vi "ESTTL.vi"(8 "error in (no error)":errorcluster, 11 "Node Ptr":T4 format="%.0x") -> (0 "error out":errorcluster)   [LabVIEW 2016, in "DCM System Explorer.lvlib"]
uses:
  DCM System Explorer.lvlib
  <vilib>/NI Veristand/Custom Device API/Custom Device Item Ref.ctl
  <vilib>/Powertrain Controls/Device Drivers/DCM/ESTTL/RT/Setup.ctl
  <vilib>/Powertrain Controls/Device Drivers/DCM/ESTTL/FPGA/Mode.ctl
  <vilib>/Powertrain Controls/Device Drivers/DCM/ESTTL/RT/Angle Control.ctl
  Shared/DCM Properties.vi
  <vilib>/NI Veristand/Custom Device API/Get Item Property (String Array).vi
  Shared/DCM Constants and GUIDs.vi
  <vilib>/NI Veristand/Custom Device API/Set Item Property (String Array).vi
  <vilib>/NI VeriStand/Custom Device API/Custom Device API.lvlib
  DCM Shared.lvlib
  <vilib>/Powertrain Controls/Device Drivers/DCM/ESTTL/RT/DCM - RT - ESTTL.lvlib
  <vilib>/Powertrain Controls/Device Drivers/DCM/ESTTL/FPGA/DCM - FPGA - ESTTL.lvlib
panel:
  in  "_Setup Element":T1={"Mode"=enum."Off", "Polarity"=FALSE, "Frequency [Hz]"=0.0, "Duty Cycle [%]"=0.0, "TDC Offset [CAD]"=0.0, "Window Start [DBTDC]"=0.0, "Window End [DBTDC]"=0.0, "Angles"=[{"Enable"=FALSE, "Location [DBTDC]"=0.0, "Duration [s]"=0.0}, {"Enable"=FALSE, "Location [DBTDC]"=0.0, "Duration [s]"=0.0}, {"Enable"=FALSE, "Location [DBTDC]"=0.0, "Duration [s]"=0.0}, {"Enable"=FALSE, "Location [DBTDC]"=0.0, "Duration [s]"=0.0}], "Skip Fire"=FALSE, "Skip Fire Index"=0} {"Skip Fire Index" max=7; "Angles"."Duration [s]" format="%#_3p"; "Frequency [Hz]" format="%#_3p"}
  in  "_Refresh":bool
  in  "Channel Names":string[](array[string])=["", "", "", "", "", "", "", "", "", "", "", ""]
  in  "Channel Name":string
  in  "_ESTTL Channels":i32[](listbox) caption="Channel Summary"
  in  "_Save Changes?":bool
  in  "Setup":T1[](array[typedef]) caption="ESTTL Setup" {"Skip Fire Index" max=7; "Angles"."Duration [s]" format="%#_3p"; "Frequency [Hz]" format="%#_3p"}
  in  "Header":cluster{"Section Name":string}={"Section Name"="ESTTL I/O Initial Settings"}
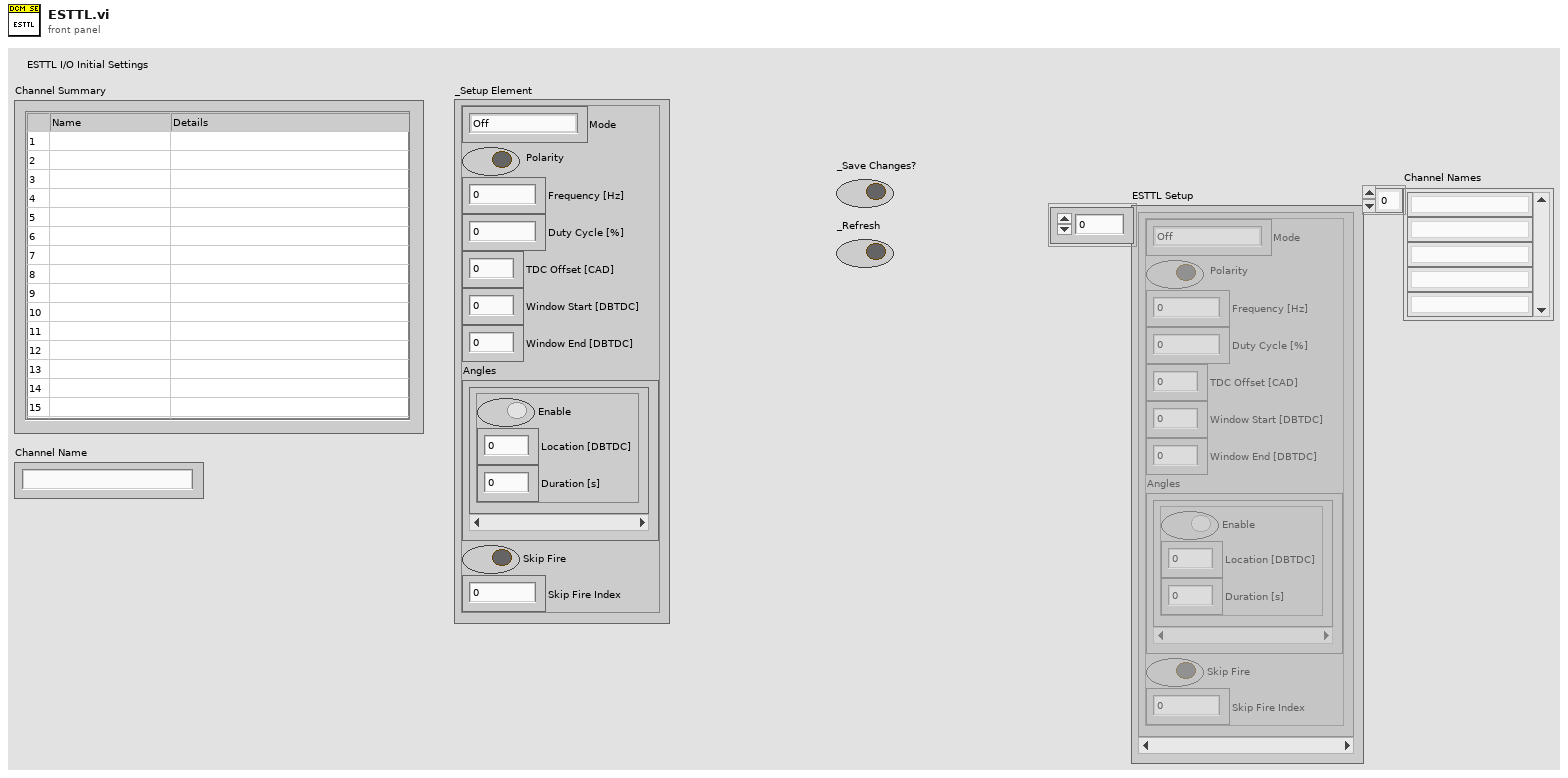
[diagram p1: front panel]
types:
  T1 = typedef "DCM - RT - ESTTL.lvlib/Setup.ctl" = cluster{"Mode":T2, "Polarity":bool, "Frequency [Hz]":sgl, "Duty Cycle [%]":sgl, "TDC Offset [CAD]":sgl, "Window Start [DBTDC]":sgl, "Window End [DBTDC]":sgl, "Angles":T3[], "Skip Fire":bool, "Skip Fire Index":u8}
  T2 = typedef "DCM - FPGA - ESTTL.lvlib/Mode.ctl" = enum8{"Off", "Pulse Width Modulation", "Engine Position Tracking"}
  T3 = typedef "DCM - RT - ESTTL.lvlib/Angle Control.ctl" = cluster{"Enable":bool, "Location [DBTDC]":sgl, "Duration [s]":sgl}
  T4 = typedef "Custom Device API.lvlib/Custom Device Item Ref.ctl" = u64
  T5 = typedef "Custom Device API.lvlib/Custom Device Commands.ctl" = enum16{"Default", "Item renamed", "Shutdown", "Dynamic button pressed"}
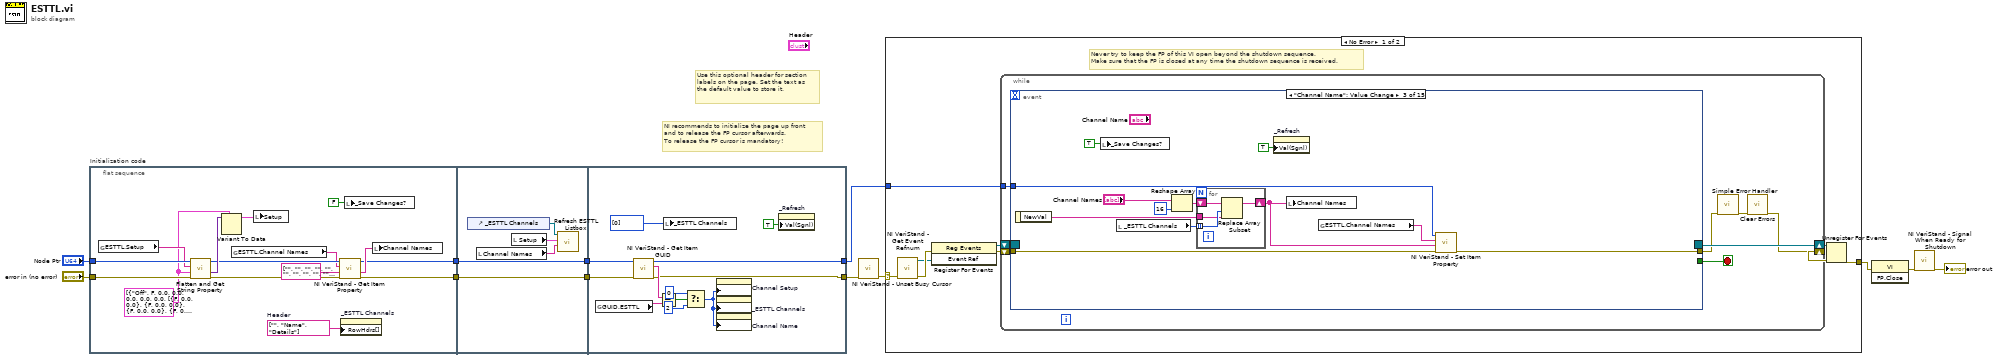
[diagram p0: block diagram]
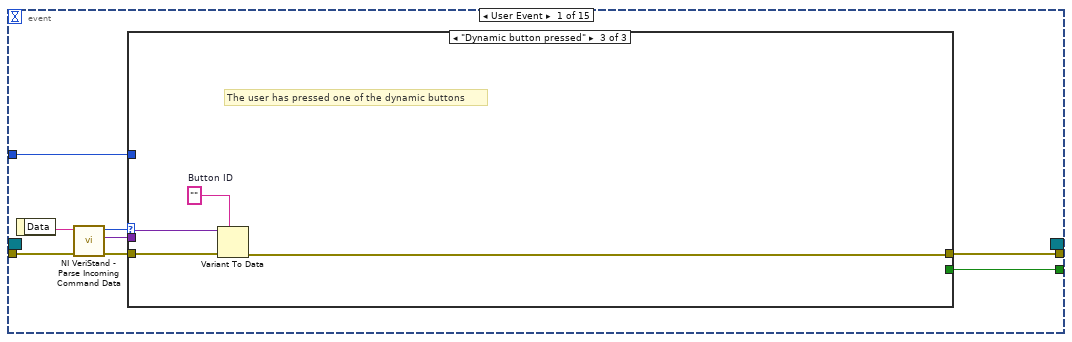
[diagram p2: hidden frame]
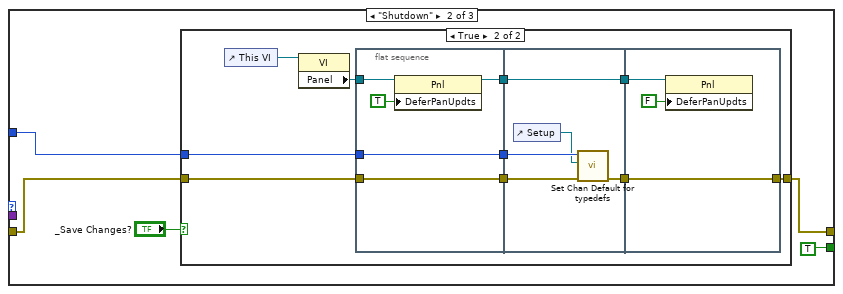
[diagram p4: hidden frame]
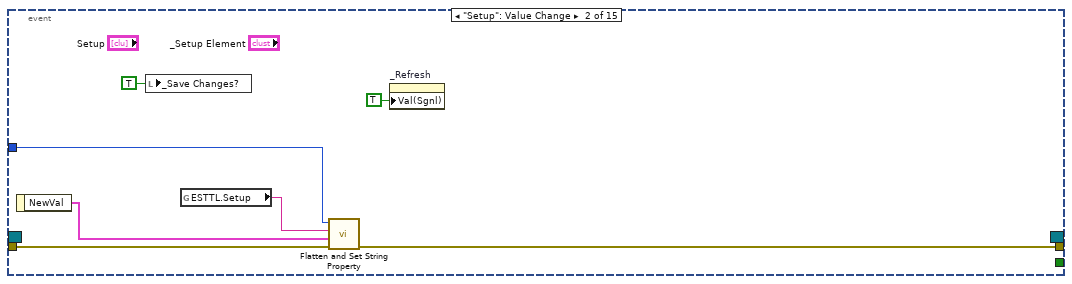
[diagram p6: hidden frame]
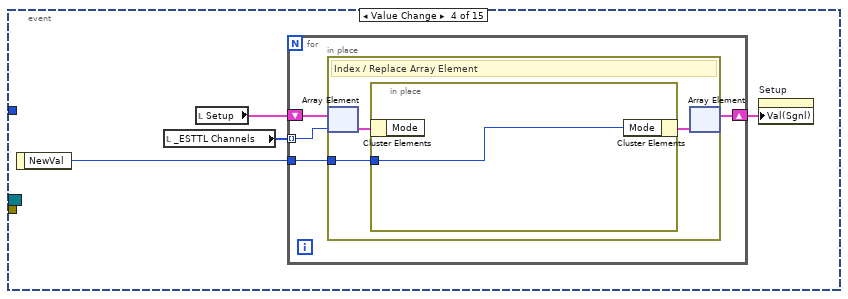
[diagram p7: hidden frame]
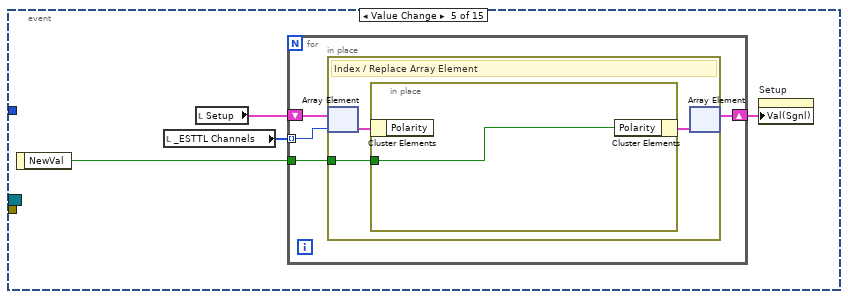
[diagram p8: hidden frame]
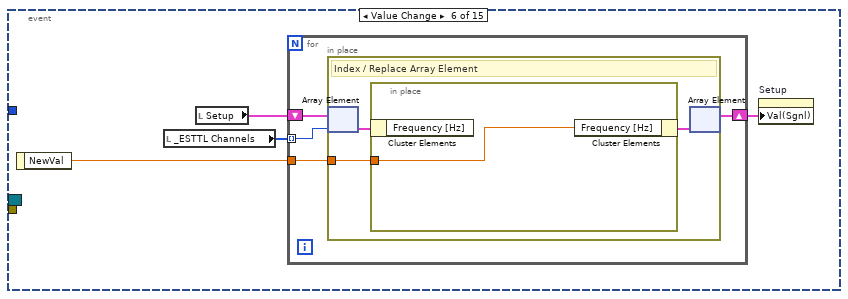
[diagram p9: hidden frame]
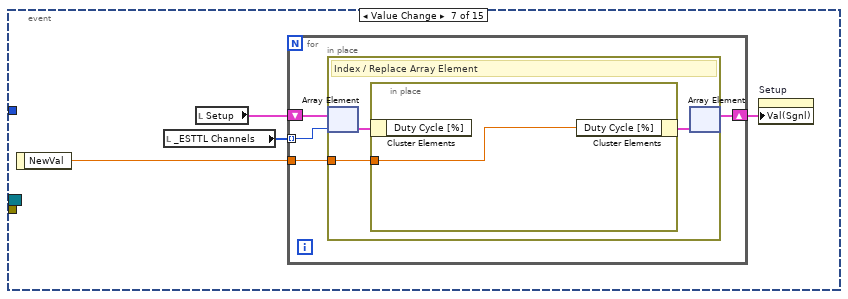
[diagram p10: hidden frame]
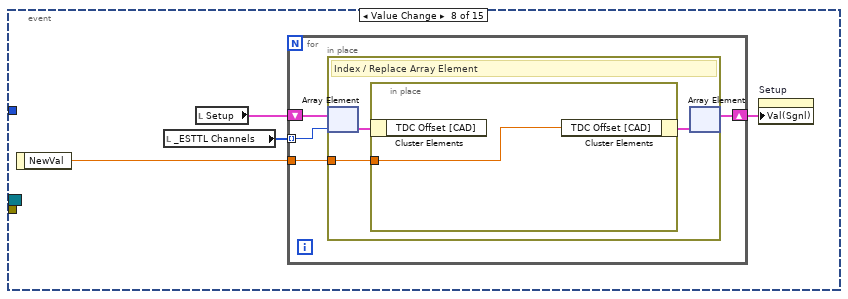
[diagram p11: hidden frame]
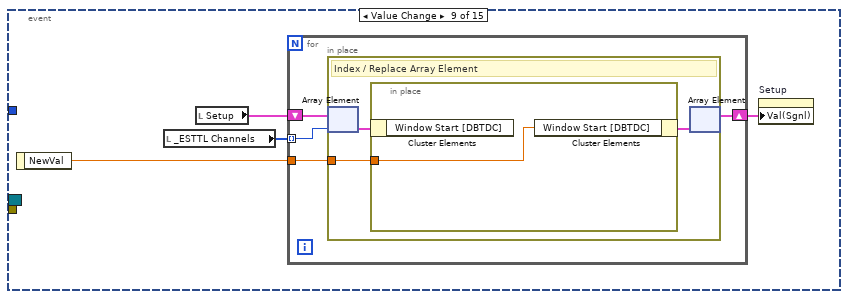
[diagram p12: hidden frame]
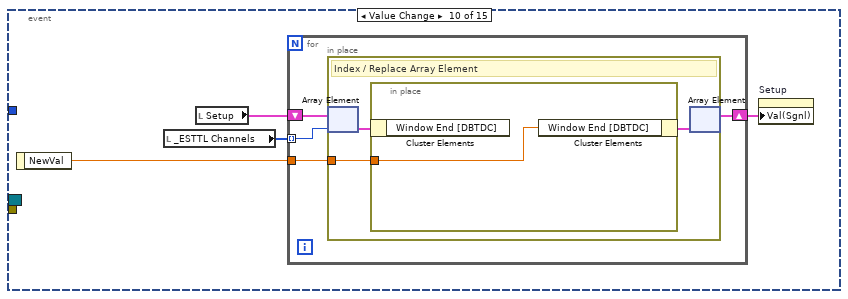
[diagram p13: hidden frame]
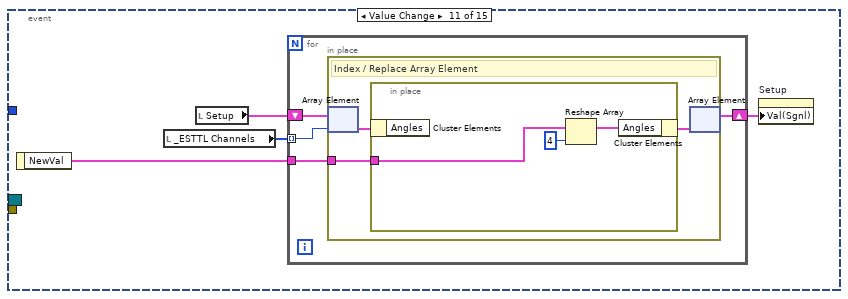
[diagram p14: hidden frame]
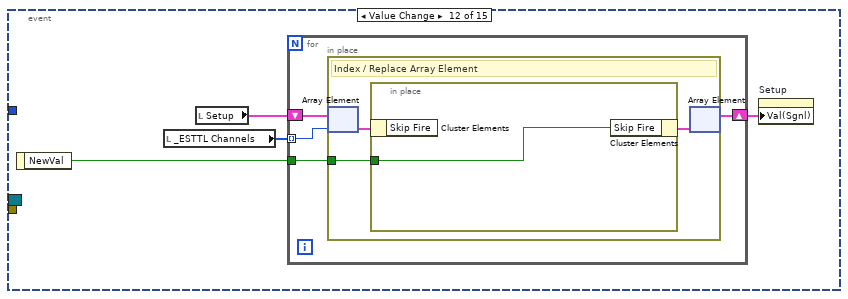
[diagram p15: hidden frame]
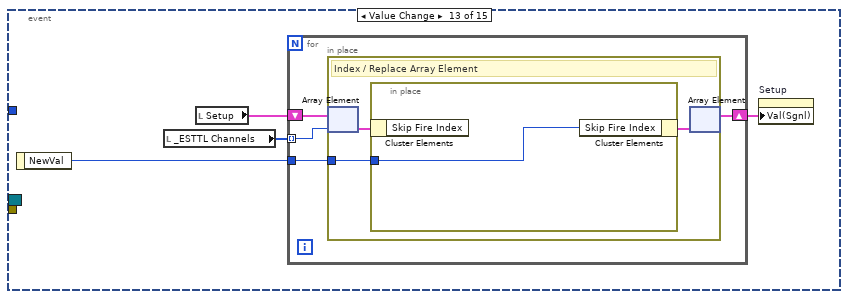
[diagram p16: hidden frame]
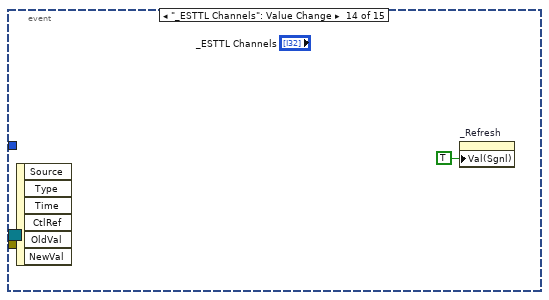
[diagram p17: hidden frame]
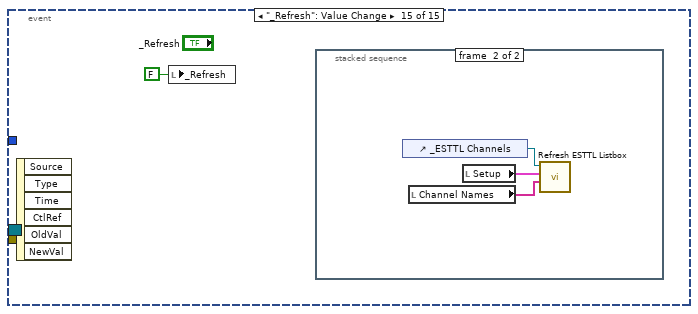
[diagram p18: hidden frame]
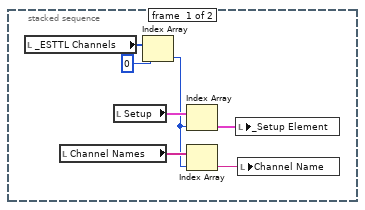
[diagram p19: hidden frame]
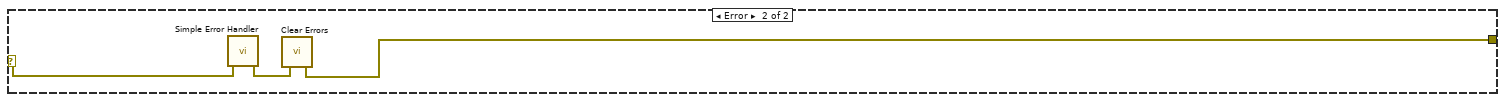
[diagram p20: hidden frame]
diagram:
  # "Use this optional header for section labels on the page. Set the text as the default value to store it."
  # "NI recommends to initialize the page up front\nand to release the FP cursor afterwards.\nTo release the FP cursor is mandatory!"
  n1 = flat-sequence "Initialization code" {
    tunnel: "Node Ptr" -> [w25]
    tunnel: "error in (no error)" -> [w26]
    tunnel: [w16] -> w5
    tunnel: [w15] -> w4
    tunnel: w5 -> [w32]
    tunnel: w4 -> [w31]
    tunnel: [w32] -> w3
    tunnel: [w31] -> w2
    tunnel: [w36] -> w1
    tunnel: [w38] -> w6
    tunnel: w3 -> [w39]
    tunnel: w2 -> [w37]
    frame #0 {
      w13 = string[] ["", "Name", "Details"]  # Header
      w23 = T1[] [{"Mode"=enum."Off", "Polarity"=FALSE, "Frequency [Hz]"=0.0, "Duty Cycle [%]"=0.0, "TDC Offset [CAD]"=0.0, "Window Start [DBTDC]"=0.0, "Window End [DBTDC]"=0.0, "Angles"=[{"Enable"=FALSE, "Location [DBTDC]"=0.0, "Duration [s]"=0.0}, {"Enable"=FALSE, "Location [DBTDC]"=0.0, "Duration [s]"=0.0}, {"Enable"=FALSE, "Location [DBTDC]"=0.0, "Duration [s]"=0.0}, {"Enable"=FALSE, "Location [DBTDC]"=0.0, "Duration [s]"=0.0}], "Skip Fire"=FALSE, "Skip Fire Index"=0}, {"Mode"=enum."Off", "Polarity"=FALSE, "Frequency [Hz]"=0.0, "Duty Cycle [%]"=0.0, "TDC Offset [CAD]"=0.0, "Window Start [DBTDC]"=0.0, "Window End [DBTDC]"=0.0, "Angles"=[{"Enable"=FALSE, "Location [DBTDC]"=0.0, "Duration [s]"=0.0}, {"Enable"=FALSE, "Location [DBTDC]"=0.0, "Duration [s]"=0.0}, {"Enable"=FALSE, "Location [DBTDC]"=0.0, "Duration [s]"=0.0}, {"Enable"=FALSE, "Location [DBTDC]"=0.0, "Duration [s]"=0.0}], "Skip Fire"=FALSE, "Skip Fire Index"=0}, {"Mode"=enum."Off", "Polarity"=FALSE, "Frequency [Hz]"=0.0, "Duty Cycle [%]"=0.0, "TDC Offset [CAD]"=0.0, "Window Start [DBTDC]"=0.0, "Window End [DBTDC]"=0.0, "Angles"=[{"Enable"=FALSE, "Location [DBTDC]"=0.0, "Duration [s]"=0.0}, {"Enable"=FALSE, "Location [DBTDC]"=0.0, "Duration [s]"=0.0}, {"Enable"=FALSE, "Location [DBTDC]"=0.0, "Duration [s]"=0.0}, {"Enable"=FALSE, "Location [DBTDC]"=0.0, "Duration [s]"=0.0}], "Skip Fire"=FALSE, "Skip Fire Index"=0}, {"Mode"=enum."Off", "Polarity"=FALSE, "Frequency [Hz]"=0.0, "Duty Cycle [%]"=0.0, "TDC Offset [CAD]"=0.0, "Window Start [DBTDC]"=0.0, "Window End [DBTDC]"=0.0, "Angles"=[{"Enable"=FALSE, "Location [DBTDC]"=0.0, "Duration [s]"=0.0}, {"Enable"=FALSE, "Location [DBTDC]"=0.0, "Duration [s]"=0.0}, {"Enable"=FALSE, "Location [DBTDC]"=0.0, "Duration [s]"=0.0}, {"Enable"=FALSE, "Location [DBTDC]"=0.0, "Duration [s]"=0.0}], "Skip Fire"=FALSE, "Skip Fire Index"=0}, {"Mode"=enum."Off", "Polarity"=FALSE, "Frequency [Hz]"=0.0, "Duty Cycle [%]"=0.0, "TDC Offset [CAD]"=0.0, "Window Start [DBTDC]"=0.0, "Window End [DBTDC]"=0.0, "Angles"=[{"Enable"=FALSE, "Location [DBTDC]"=0.0, "Duration [s]"=0.0}, {"Enable"=FALSE, "Location [DBTDC]"=0.0, "Duration [s]"=0.0}, {"Enable"=FALSE, "Location [DBTDC]"=0.0, "Duration [s]"=0.0}, {"Enable"=FALSE, "Location [DBTDC]"=0.0, "Duration [s]"=0.0}], "Skip Fire"=FALSE, "Skip Fire Index"=0}, {"Mode"=enum."Off", "Polarity"=FALSE, "Frequency [Hz]"=0.0, "Duty Cycle [%]"=0.0, "TDC Offset [CAD]"=0.0, "Window Start [DBTDC]"=0.0, "Window End [DBTDC]"=0.0, "Angles"=[{"Enable"=FALSE, "Location [DBTDC]"=0.0, "Duration [s]"=0.0}, {"Enable"=FALSE, "Location [DBTDC]"=0.0, "Duration [s]"=0.0}, {"Enable"=FALSE, "Location [DBTDC]"=0.0, "Duration [s]"=0.0}, {"Enable"=FALSE, "Location [DBTDC]"=0.0, "Duration [s]"=0.0}], "Skip Fire"=FALSE, "Skip Fire Index"=0}, {"Mode"=enum."Off", "Polarity"=FALSE, "Frequency [Hz]"=0.0, "Duty Cycle [%]"=0.0, "TDC Offset [CAD]"=0.0, "Window Start [DBTDC]"=0.0, "Window End [DBTDC]"=0.0, "Angles"=[{"Enable"=FALSE, "Location [DBTDC]"=0.0, "Duration [s]"=0.0}, {"Enable"=FALSE, "Location [DBTDC]"=0.0, "Duration [s]"=0.0}, {"Enable"=FALSE, "Location [DBTDC]"=0.0, "Duration [s]"=0.0}, {"Enable"=FALSE, "Location [DBTDC]"=0.0, "Duration [s]"=0.0}], "Skip Fire"=FALSE, "Skip Fire Index"=0}, {"Mode"=enum."Off", "Polarity"=FALSE, "Frequency [Hz]"=0.0, "Duty Cycle [%]"=0.0, "TDC Offset [CAD]"=0.0, "Window Start [DBTDC]"=0.0, "Window End [DBTDC]"=0.0, "Angles"=[{"Enable"=FALSE, "Location [DBTDC]"=0.0, "Duration [s]"=0.0}, {"Enable"=FALSE, "Location [DBTDC]"=0.0, "Duration [s]"=0.0}, {"Enable"=FALSE, "Location [DBTDC]"=0.0, "Duration [s]"=0.0}, {"Enable"=FALSE, "Location [DBTDC]"=0.0, "Duration [s]"=0.0}], "Skip Fire"=FALSE, "Skip Fire Index"=0}] ("DiffIO.Setup")
      n2 = global read "DCM Properties.vi" "ESTTL.Setup"() -> (w24:string)
      n3 = call "Flatten and Get String Property.vi"("error in (no error)"=w26, "Default Value"=w23, "Property Name"=w24, "Section Ref in"=w25) -> ("error out"=w20:errorcluster, "Value"=w27:variant, "Section Ref out"=w21:T4)  [unwired: 5 in]
      n4 = Variant To Data(type=w23, Variant=w27) -> (data=w22:T1[])  [unwired: 1 in, 1 out]
      n5 = global read "DCM Properties.vi" "ESTTL.Channel Names"() -> (w18:string)
      n6 = local write "Setup"(w22) -> ()
      n7 = call-poly <vilib>:"NI VeriStand - Get Item Property.vi"("error in (no error)"=w20, "Default Value"=string[] ["", "", "", "", "", "", "", "", "", "", "", "", "", "", "", ""], "Property Name"=w18, "Item Ref in"=w21) -> ("error out"=w15:errorcluster, "Value"=w17:string[], "Item Ref out"=w16:T4)  [unwired: 4 in, 1 out]
      n8 = property on="_ESTTL Channels" class="MCListbox (strict)"("RowHdrs[]"=w13) -> ()  [unwired: 2 in, 2 out]
      n9 = local write "_Save Changes?"(FALSE ("_Save Changes?")) -> ()
      n10 = local write "Channel Names"(w17) -> ()
    }
    frame #1 {
      n11 = control-ref of="_ESTTL Channels"() -> (w28:refnum<vi>)
      n12 = local read "Channel Names"() -> (w30:string[])
      n13 = local read "Setup"() -> (w29:T1[])
      n14 = call "Refresh ESTTL Listbox.vi"("Names"=w30, "Setup"=w29, "MulticolumnListbox in"=w28) -> ()  [unwired: 9 in]
    }
    frame #2 {
      n15 = global read "DCM Constants and GUIDs.vi" "GUID.ESTTL"() -> (w40:string)
      n16 = call <vilib>:"NI VeriStand - Get Item GUID.vi"("error in (no error)"=w37, "Item Ref in"=w39) -> ("error out"=w36:errorcluster, "GUID"=w41:string, "Item Ref out"=w38:T4)  [unwired: 7 in]
      n17 = Equal?(x=w41, y=w40) -> (x = y?=w35:bool)
      n18 = local write "_ESTTL Channels"(i32[] [0] ("Channel Setup Summary")) -> ()
      n19 = Select(t=0, s=w35, f=2) -> (s? t:f=w44:i32)
      n20 = property on="Channel Setup" class="Clust (strict)"("DisabledEnum"=w44) -> ()  [unwired: 2 in, 2 out]
      n21 = property on="_ESTTL Channels" class="MCListbox (strict)"("DisabledEnum"=w44) -> ()  [unwired: 2 in, 2 out]
      n22 = property on="Channel Name" class="Str"("DisabledEnum"=w44) -> ()  [unwired: 2 in, 2 out]
      n23 = property on="_Refresh" class="Bool (strict)"("Val(Sgnl)"=TRUE ("_Refresh")) -> ()  [unwired: 2 in, 2 out]
    }
  }
  n24 = call <vilib>:"NI VeriStand - Unset Busy Cursor.vi"("error in (no error)"=w1) -> ("error out"=w8:errorcluster)  [unwired: 10 out]
  n25 = case shown="No Error" w8 {
    selector: w8 -> [w46 w263]
    tunnel: [w50 w261] -> w12
    tunnel: w6 -> [w45 _]
    frame No Error {
      # "Never try to keep the FP of this VI open beyond the shutdown sequence.\nMake sure that the FP is closed at any time the shutdown sequence is received."
      n26 = call <vilib>:"NI VeriStand - Get Event Refnum.vi"("error in (no error)"=w46) -> ("error out"=w53:errorcluster, "Event Ref"=w49:refnum<user-event>)  [unwired: 9 out]
      n27 = register-events(error in=w53, w49) -> (reference out=w47:refnum<event-registration>, error out=w48:errorcluster)  [unwired: 1 in]
      n28 = while {
        shift-right: [w55] -> w51
        shift-left: w48 -> [w60]
        shift-right: [w61] -> w52
        shift-left: w47 -> [w59]
        tunnel: w45 -> [w54]
        stop <- w58 stop-if-true
        n29 = event shown="[2] \"Channel Name\": Value Change" {
          selector: w59 -> [_ _ _ _ _ _ _ _ _ _ _ _ _ _ _]
          dyn-events: [_ _ _ _ _ _ _ _ _ _ _ _ _ _ _] -> w61
          timeout: _ -> [_ _ _ _ _ _ _ _ _ _ _ _ _ _ _]
          tunnel: w60 -> [w69 w110 w122 _ _ _ _ _ _ _ _ _ _ _ _]
          tunnel: [w65 _ _ _ _ _ _ _ _ _ _ _ _ _ _] -> w58
          tunnel: [w64 w109 w121 _ _ _ _ _ _ _ _ _ _ _ _] -> w57
          tunnel: w54 -> [w62 w106 w119 _ _ _ _ _ _ _ _ _ _ _ _]
          event User Event {
            n30 = event-data() -> ("Data"=w68:string)  [unwired: 1 out]
            n31 = call <vilib>:"NI VeriStand - Parse Incoming Command Data.vi"("error in (no error)"=w69, "Incoming data"=w68) -> ("error out"=w67:errorcluster, "Outgoing data"=w63:variant, "Action"=w66:T5)  [unwired: 7 out]
            n32 = case shown="\"Dynamic button pressed\"" w66 {
              tunnel: w67 -> [w70 w73 w103]
              tunnel: [_ TRUE _] -> w65
              tunnel: [w70 w72 w100] -> w64
              tunnel: w63 -> [_ _ w102]
              tunnel: w62 -> [_ w74 _]
              frame "Default", Default {
              }
              frame "Shutdown" {
                n33 = case shown="True" "_Save Changes?" {
                  tunnel: w74 -> [_ w81]
                  tunnel: w73 -> [w76 w80]
                  tunnel: [w76 w79] -> w72
                  frame False {
                  }
                  frame True {
                    n34 = control-ref of="This VI"() -> (w78:refnum<vi>)
                    n35 = property class="VI"(reference=w78) -> ("Panel"=w77:refnum<vi>)  [unwired: 1 in, 2 out]
                    n36 = flat-sequence {
                      tunnel: w80 -> [w90]
                      tunnel: w81 -> [w91]
                      tunnel: [w91] -> w86
                      tunnel: [w90] -> w85
                      tunnel: w77 -> [w89]
                      tunnel: [w87] -> w84
                      tunnel: w86 -> [w96]
                      tunnel: w85 -> [w95]
                      tunnel: [w94] -> w83
                      tunnel: [w93] -> w82
                      tunnel: w84 -> [w93]
                      tunnel: [w99] -> w79
                      tunnel: w83 -> [w99]
                      tunnel: w82 -> [w97]
                      frame #0 {
                        n37 = property class="Pnl"(reference=w89, "DeferPanUpdts"=TRUE ("Defer Panel Updates")) -> (reference out=w87:refnum<vi>)  [unwired: 1 in, 1 out]
                      }
                      frame #1 {
                        n38 = control-ref of="Setup"() -> (w92:refnum<vi>)
                        n39 = call "Set Chan Default for typedefs.vi"("error in"=w95, "Ctl Ref"=w92, "Section Ref in"=w96) -> ("error out"=w94:errorcluster)  [unwired: 7 in, 1 out]
                      }
                      frame #2 {
                        n40 = property class="Pnl"(reference=w97, "DeferPanUpdts"=FALSE ("Defer Panel Updates")) -> ()  [unwired: 1 in, 2 out]
                      }
                    }
                  }
                }
              }
              frame "Dynamic button pressed" {
                w101 = ""  # Button ID
                # "The user has pressed one of the dynamic buttons"
                n41 = Variant To Data(error in=w103, type=w101, Variant=w102) -> (error out=w100:errorcluster)  [unwired: 1 out]
              }
            }
          }
          event "Setup": Value Change {
            n42 = event-data() -> ("NewVal"=w107:T1[])  [unwired: 1 out]
            n43 = local write "_Save Changes?"(TRUE ("_Save Changes?")) -> ()
            n44 = global read "DCM Properties.vi" "ESTTL.Setup"() -> (w108:string)
            n45 = call "Flatten and Set String Property.vi"("error in (no error)"=w110, "Value"=w107, "Property Name"=w108, "Section Ref in"=w106) -> ("error out"=w109:errorcluster)  [unwired: 6 in, 1 out]
            n46 = property on="_Refresh" class="Bool (strict)"("Val(Sgnl)"=TRUE ("_Refresh")) -> ()  [unwired: 2 in, 2 out]
          }
          event "Channel Name": Value Change {
            n47 = event-data() -> ("NewVal"=w113:string)  [unwired: 1 out]
            n48 = local write "_Save Changes?"(TRUE ("_Save Changes?")) -> ()
            n49 = local read "_ESTTL Channels"() -> (w115:i32[])
            n50 = Reshape Array("Channel Names", 16 ("dimension size")) -> (w117:string[])
            n51 = for {
              tunnel: w115 -> [w124] mode=indexing
              shift-right: [w125] -> w111
              shift-left: w117 -> [w126]
              tunnel: w113 -> [w123]
              n52 = Replace Array Subset(array=w126, new element=w123, index=w124) -> (w125:string[])
            }
            n53 = property on="_Refresh" class="Bool (strict)"("Val(Sgnl)"=TRUE ("_Refresh")) -> ()  [unwired: 2 in, 2 out]
            n54 = local write "Channel Names"(w111) -> ()
            n55 = global read "DCM Properties.vi" "ESTTL.Channel Names"() -> (w120:string)
            n56 = call-poly <vilib>:"NI VeriStand - Set Item Property.vi"("error in (no error)"=w122, "Value"=w111, "Property Name"=w120, "Item Ref in"=w119) -> ("error out"=w121:errorcluster)  [unwired: 5 in, 2 out]
          }
          event Value Change {
            n57 = event-data() -> ("NewVal"=w127:T2)  [unwired: 1 out]
            n58 = local read "_ESTTL Channels"() -> (w128:i32[])
            n59 = local read "Setup"() -> (w129:T1[])
            n60 = for {
              tunnel: w128 -> [w133] mode=indexing
              shift-right: [w132] -> w130
              shift-left: w129 -> [w134]
              tunnel: w127 -> [w131]
              n61 = in-place {
                in-place-border: w131 -> [w135]
                # "Index / Replace Array Element"
                n62 = in-place-array #1(w134, w133) -> (w137:T1)
                n63 = in-place {
                  in-place-border: w135 -> [w138]
                  n64 = in-place-cluster #2(w137) -> ()  [unwired: 1 out]
                  n65 = in-place-cluster #2("Mode"=w138) -> (w136:T1)
                }
                n66 = in-place-array #1(w136) -> (w132:T1[])  [unwired: 1 out]
              }
            }
            n67 = property on="Setup" class="Arr (strict)"("Val(Sgnl)"=w130) -> ()  [unwired: 2 in, 2 out]
          }
          event Value Change {
            n68 = event-data() -> ("NewVal"=w139:bool)  [unwired: 1 out]
            n69 = local read "_ESTTL Channels"() -> (w140:i32[])
            n70 = local read "Setup"() -> (w141:T1[])
            n71 = for {
              tunnel: w140 -> [w145] mode=indexing
              shift-right: [w144] -> w142
              shift-left: w141 -> [w146]
              tunnel: w139 -> [w143]
              n72 = in-place {
                in-place-border: w143 -> [w147]
                # "Index / Replace Array Element"
                n73 = in-place-array #3(w146, w145) -> (w149:T1)
                n74 = in-place {
                  in-place-border: w147 -> [w150]
                  n75 = in-place-cluster #4(w149) -> ()  [unwired: 1 out]
                  n76 = in-place-cluster #4("Polarity"=w150) -> (w148:T1)
                }
                n77 = in-place-array #3(w148) -> (w144:T1[])  [unwired: 1 out]
              }
            }
            n78 = property on="Setup" class="Arr (strict)"("Val(Sgnl)"=w142) -> ()  [unwired: 2 in, 2 out]
          }
          event Value Change {
            n79 = event-data() -> ("NewVal"=w151:sgl)  [unwired: 1 out]
            n80 = local read "_ESTTL Channels"() -> (w152:i32[])
            n81 = local read "Setup"() -> (w153:T1[])
            n82 = for {
              tunnel: w152 -> [w157] mode=indexing
              shift-right: [w156] -> w154
              shift-left: w153 -> [w158]
              tunnel: w151 -> [w155]
              n83 = in-place {
                in-place-border: w155 -> [w159]
                # "Index / Replace Array Element"
                n84 = in-place-array #5(w158, w157) -> (w161:T1)
                n85 = in-place {
                  in-place-border: w159 -> [w162]
                  n86 = in-place-cluster #6(w161) -> ()  [unwired: 1 out]
                  n87 = in-place-cluster #6("Frequency [Hz]"=w162) -> (w160:T1)
                }
                n88 = in-place-array #5(w160) -> (w156:T1[])  [unwired: 1 out]
              }
            }
            n89 = property on="Setup" class="Arr (strict)"("Val(Sgnl)"=w154) -> ()  [unwired: 2 in, 2 out]
          }
          event Value Change {
            n90 = event-data() -> ("NewVal"=w163:sgl)  [unwired: 1 out]
            n91 = local read "_ESTTL Channels"() -> (w164:i32[])
            n92 = local read "Setup"() -> (w165:T1[])
            n93 = for {
              tunnel: w164 -> [w169] mode=indexing
              shift-right: [w168] -> w166
              shift-left: w165 -> [w170]
              tunnel: w163 -> [w167]
              n94 = in-place {
                in-place-border: w167 -> [w171]
                # "Index / Replace Array Element"
                n95 = in-place-array #7(w170, w169) -> (w173:T1)
                n96 = in-place {
                  in-place-border: w171 -> [w174]
                  n97 = in-place-cluster #8(w173) -> ()  [unwired: 1 out]
                  n98 = in-place-cluster #8("Duty Cycle [%]"=w174) -> (w172:T1)
                }
                n99 = in-place-array #7(w172) -> (w168:T1[])  [unwired: 1 out]
              }
            }
            n100 = property on="Setup" class="Arr (strict)"("Val(Sgnl)"=w166) -> ()  [unwired: 2 in, 2 out]
          }
          event Value Change {
            n101 = event-data() -> ("NewVal"=w175:sgl)  [unwired: 1 out]
            n102 = local read "_ESTTL Channels"() -> (w176:i32[])
            n103 = local read "Setup"() -> (w177:T1[])
            n104 = for {
              tunnel: w176 -> [w181] mode=indexing
              shift-right: [w180] -> w178
              shift-left: w177 -> [w182]
              tunnel: w175 -> [w179]
              n105 = in-place {
                in-place-border: w179 -> [w183]
                # "Index / Replace Array Element"
                n106 = in-place-array #9(w182, w181) -> (w185:T1)
                n107 = in-place {
                  in-place-border: w183 -> [w186]
                  n108 = in-place-cluster #10(w185) -> ()  [unwired: 1 out]
                  n109 = in-place-cluster #10("TDC Offset [CAD]"=w186) -> (w184:T1)
                }
                n110 = in-place-array #9(w184) -> (w180:T1[])  [unwired: 1 out]
              }
            }
            n111 = property on="Setup" class="Arr (strict)"("Val(Sgnl)"=w178) -> ()  [unwired: 2 in, 2 out]
          }
          event Value Change {
            n112 = event-data() -> ("NewVal"=w187:sgl)  [unwired: 1 out]
            n113 = local read "_ESTTL Channels"() -> (w188:i32[])
            n114 = local read "Setup"() -> (w189:T1[])
            n115 = for {
              tunnel: w188 -> [w193] mode=indexing
              shift-right: [w192] -> w190
              shift-left: w189 -> [w194]
              tunnel: w187 -> [w191]
              n116 = in-place {
                in-place-border: w191 -> [w195]
                # "Index / Replace Array Element"
                n117 = in-place-array #11(w194, w193) -> (w197:T1)
                n118 = in-place {
                  in-place-border: w195 -> [w198]
                  n119 = in-place-cluster #12(w197) -> ()  [unwired: 1 out]
                  n120 = in-place-cluster #12("Window Start [DBTDC]"=w198) -> (w196:T1)
                }
                n121 = in-place-array #11(w196) -> (w192:T1[])  [unwired: 1 out]
              }
            }
            n122 = property on="Setup" class="Arr (strict)"("Val(Sgnl)"=w190) -> ()  [unwired: 2 in, 2 out]
          }
          event Value Change {
            n123 = event-data() -> ("NewVal"=w199:sgl)  [unwired: 1 out]
            n124 = local read "_ESTTL Channels"() -> (w200:i32[])
            n125 = local read "Setup"() -> (w201:T1[])
            n126 = for {
              tunnel: w200 -> [w205] mode=indexing
              shift-right: [w204] -> w202
              shift-left: w201 -> [w206]
              tunnel: w199 -> [w203]
              n127 = in-place {
                in-place-border: w203 -> [w207]
                # "Index / Replace Array Element"
                n128 = in-place-array #13(w206, w205) -> (w209:T1)
                n129 = in-place {
                  in-place-border: w207 -> [w210]
                  n130 = in-place-cluster #14(w209) -> ()  [unwired: 1 out]
                  n131 = in-place-cluster #14("Window End [DBTDC]"=w210) -> (w208:T1)
                }
                n132 = in-place-array #13(w208) -> (w204:T1[])  [unwired: 1 out]
              }
            }
            n133 = property on="Setup" class="Arr (strict)"("Val(Sgnl)"=w202) -> ()  [unwired: 2 in, 2 out]
          }
          event Value Change {
            n134 = event-data() -> ("NewVal"=w211:T3[])  [unwired: 1 out]
            n135 = local read "_ESTTL Channels"() -> (w212:i32[])
            n136 = local read "Setup"() -> (w213:T1[])
            n137 = for {
              tunnel: w212 -> [w217] mode=indexing
              shift-right: [w216] -> w214
              shift-left: w213 -> [w218]
              tunnel: w211 -> [w215]
              n138 = in-place {
                in-place-border: w215 -> [w219]
                # "Index / Replace Array Element"
                n139 = in-place-array #15(w218, w217) -> (w221:T1)
                n140 = in-place {
                  in-place-border: w219 -> [w224]
                  n141 = in-place-cluster #16(w221) -> ()  [unwired: 1 out]
                  n142 = Reshape Array(w224, 4 ("dimension size")) -> (w223:T3[])
                  n143 = in-place-cluster #16("Angles"=w223) -> (w220:T1)
                }
                n144 = in-place-array #15(w220) -> (w216:T1[])  [unwired: 1 out]
              }
            }
            n145 = property on="Setup" class="Arr (strict)"("Val(Sgnl)"=w214) -> ()  [unwired: 2 in, 2 out]
          }
          event Value Change {
            n146 = event-data() -> ("NewVal"=w225:bool)  [unwired: 1 out]
            n147 = local read "_ESTTL Channels"() -> (w226:i32[])
            n148 = local read "Setup"() -> (w227:T1[])
            n149 = for {
              tunnel: w226 -> [w231] mode=indexing
              shift-right: [w230] -> w228
              shift-left: w227 -> [w232]
              tunnel: w225 -> [w229]
              n150 = in-place {
                in-place-border: w229 -> [w233]
                # "Index / Replace Array Element"
                n151 = in-place-array #17(w232, w231) -> (w235:T1)
                n152 = in-place {
                  in-place-border: w233 -> [w236]
                  n153 = in-place-cluster #18(w235) -> ()  [unwired: 1 out]
                  n154 = in-place-cluster #18("Skip Fire"=w236) -> (w234:T1)
                }
                n155 = in-place-array #17(w234) -> (w230:T1[])  [unwired: 1 out]
              }
            }
            n156 = property on="Setup" class="Arr (strict)"("Val(Sgnl)"=w228) -> ()  [unwired: 2 in, 2 out]
          }
          event Value Change {
            n157 = event-data() -> ("NewVal"=w237:u8)  [unwired: 1 out]
            n158 = local read "_ESTTL Channels"() -> (w238:i32[])
            n159 = local read "Setup"() -> (w239:T1[])
            n160 = for {
              tunnel: w238 -> [w243] mode=indexing
              shift-right: [w242] -> w240
              shift-left: w239 -> [w244]
              tunnel: w237 -> [w241]
              n161 = in-place {
                in-place-border: w241 -> [w245]
                # "Index / Replace Array Element"
                n162 = in-place-array #19(w244, w243) -> (w247:T1)
                n163 = in-place {
                  in-place-border: w245 -> [w248]
                  n164 = in-place-cluster #20(w247) -> ()  [unwired: 1 out]
                  n165 = in-place-cluster #20("Skip Fire Index"=w248) -> (w246:T1)
                }
                n166 = in-place-array #19(w246) -> (w242:T1[])  [unwired: 1 out]
              }
            }
            n167 = property on="Setup" class="Arr (strict)"("Val(Sgnl)"=w240) -> ()  [unwired: 2 in, 2 out]
          }
          event "_ESTTL Channels": Value Change {
            n168 = event-data() -> ()  [unwired: 7 out]
            n169 = property on="_Refresh" class="Bool (strict)"("Val(Sgnl)"=TRUE ("_Refresh")) -> ()  [unwired: 2 in, 2 out]
          }
          event "_Refresh": Value Change {
            n170 = event-data() -> ()  [unwired: 7 out]
            n171 = local write "_Refresh"(FALSE ("_Refresh")) -> ()
            n172 = stacked-sequence {
              frame #0 {
                n173 = local read "_ESTTL Channels"() -> (w253:i32[])
                n174 = local read "Channel Names"() -> (w257:string[])
                n175 = local read "Setup"() -> (w255:T1[])
                n176 = Index Array(array=w253, index=0) -> (element=w252:i32)
                n177 = Index Array(array=w255, index=w252) -> (element=w254:T1)
                n178 = Index Array(array=w257, index=w252) -> (element=w256:string)
                n179 = local write "_Setup Element"(w254) -> ()
                n180 = local write "Channel Name"(w256) -> ()
              }
              frame #1 {
                n181 = control-ref of="_ESTTL Channels"() -> (w260:refnum<vi>)
                n182 = local read "Channel Names"() -> (w259:string[])
                n183 = local read "Setup"() -> (w258:T1[])
                n184 = call "Refresh ESTTL Listbox.vi"("Names"=w259, "Setup"=w258, "MulticolumnListbox in"=w260) -> ()  [unwired: 9 in]
              }
            }
          }
        }
        n185 = call <vilib>:"Simple Error Handler.vi"("error in (no error)"=w57) -> ("error out"=w56:errorcluster)  [unwired: 1 in, 7 out]
        n186 = call <vilib>:"Clear Errors.vi"("error in (no error)"=w56) -> ("error out"=w55:errorcluster)  [unwired: 1 in, 5 out]
      }
      n187 = Unregister For Events(event registration refnum=w52, error in=w51) -> (error out=w50:errorcluster)
    }
    frame Error {
      n188 = call <vilib>:"Simple Error Handler.vi"("error in (no error)"=w263) -> ("error out"=w262:errorcluster)  [unwired: 1 in, 7 out]
      n189 = call <vilib>:"Clear Errors.vi"("error in (no error)"=w262) -> ("error out"=w261:errorcluster)  [unwired: 1 in, 5 out]
    }
  }
  n190 = invoke class="VI" method="FP.Close"(error in=w12) -> (error out=w11:errorcluster)  [unwired: 2 in, 2 out]
  n191 = call <vilib>:"NI VeriStand - Signal When Ready for Shutdown.vi"("error in (no error)"=w11) -> ("error out"=→"error out":errorcluster)  [unwired: 10 out]
